vi "Actor Core.vi"(8 "error in":errorcluster, 11 "SpectrometerUI in":refnum<class "SpectrometerUI.lvclass">) -> (0 "error out":errorcluster, 3 "Actor out":refnum<class "Actor.lvclass">)   [LabVIEW 2023, in "SpectrometerUI.lvlib" / "SpectrometerUI.lvclass"]
doc: "(<B>Filename</B>: Actor Framework.lvlib:Actor.lvclass:Actor Core.vi)\n\nReceives messages to the actor, reacts to them, and initiates any error handling that may shut the actor down.\n\nDescendant classes may override this VI to append parallel tasks for the actor to complete while it handles messages. Overrides use the Call Parent Class Method node."
uses:
  SpectrometerUI.lvclass
  <vilib>/ActorFramework/Actor/Actor.lvclass
  SpectrometerUI.lvclass/SpectrometerUI.ctl
panel:
  out "Wavelength Out":dbl
  in  "Set Wavelength":bool
  in  "Wavelength In":dbl
  in  "Front/Side Out":bool
  in  "Front/Side In":bool
  in  "Mirror":enum16{"Entrance Mirror", "Exit Mirror"}(ring)
  in  "Set Mirror Pos":bool
  in  "Slit":T1(ring)
  in  "Set Slitwidth":bool
  in  "Slitwidth In":dbl
  out "Slitwidth Out":dbl
  in  "Connect":bool
  in  "VISA resource name":refnum<visa-resource-name>
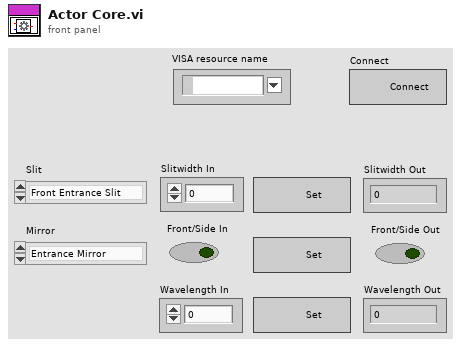
[diagram p1: front panel]
types:
  T1 = enum16{"Front Entrance Slit", "Side Entrance Slit", "Front Exit Slit", "Side Exit Slit"}
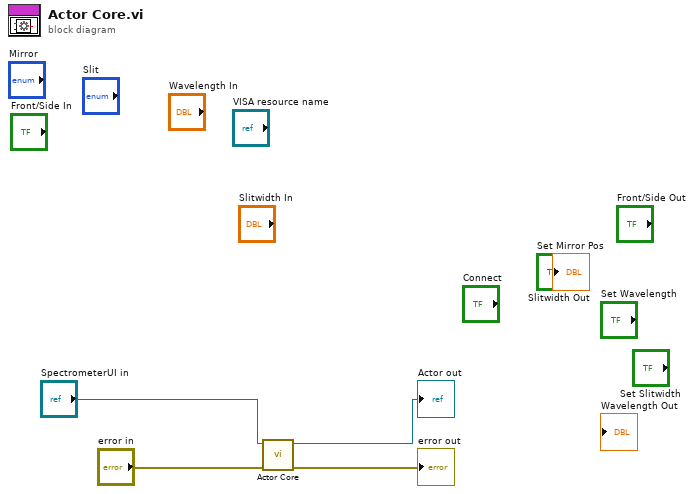
[diagram p0: block diagram]
diagram:
  n1 = call-parent "Actor Core.vi"("error in"="error in", "Actor in"="SpectrometerUI in") -> ("error out"=→"error out":errorcluster, "Actor out"=→"Actor out":refnum<class "Actor.lvclass">)  [unwired: 8 in]
